vi "SVFA Zoom Coherent Output Power.vi"(0 "scaled signal X [EUx]":waveform(dbl)={"t0"=timestamp(0 s since 1904-01-01), "dt"=1e-05, "Y"=[]}, 1 "scaled signal Y [EUy]":waveform(dbl)={"t0"=timestamp(0 s since 1904-01-01), "dt"=1e-05, "Y"=[]}, 3 "zoom settings":T8={"frequency range"={"start frequency"=1000.0, "stop frequency"=2000.0}, "window"=1, "number of lines"=400, "% overlap"=0.0} {"% overlap" min=0.0 format="%.2f"; "number of lines" min=2; "window" items=["None ", "Hanning", "Hamming", "Blackman-Harris", "Exact Blackman", "Blackman", "Flat Top", "4 Term B-Harris ", "7 Term B-Harris", "Low Sidelobe"]; "frequency range"."stop frequency" min=0.0 format="%.2f"; "frequency range"."start frequency" min=0.0 format="%.2f"}, 4 "dB On (T)":bool=TRUE, 5 "error in (no error)":errorcluster, 7 "averaging parameters":T7={"averaging mode"=enum."No averaging", "weighting mode"=enum."Exponential", "number of averages"=10, "linear mode"=enum."One shot"} {"number of averages" min=1 step=1}, 9 "restart averaging (F)":bool) -> (10 "new spectrum available":bool, 11 "averaging done":bool, 12 "coherence":cluster{"f0":dbl, "df":dbl, "coherence":dbl[]} {"coherence" format="%.2p"; "df" format="%.2p"; "f0" format="%.2p"}, 13 "averages completed":dbl, 14 "coherent output power [dB EUy]":cluster{"f0":dbl, "df":dbl, "magnitude":dbl[]} {"magnitude" format="%.2p"; "df" format="%.2p"; "f0" format="%.2p"}, 15 "unit label":string, 18 "spectrum info":T1={"channel name"="", "description"="", "x-axis units"=1, "spectral info"={"spectrum type"=enum."Power [Magnitude^2]", "linear/dB"=enum."linear", "window"=0, "window size"=0, "FFT size"=0}, "engineering units"=0, "custom label"="", "dB reference [EU]"=0.0, "peak units"=enum."rms", "weighting filter"=0, "spectral density?"=FALSE, "unit label"="", "spectrum skewed?"=FALSE, "complimentary spectrum units"=enum."none"} {"x-axis units" items=["Time (s)"=0, "Frequency-CB (Hz)"=1, "Frequency-CPB (Hz)"=1248, "Frequency-Arbitrary (Hz)"=2357, "Quefrency (s)"=2, "Revolutions (rev)"=3, "Order"=4, "Speed (RPM)"=11, "Speed (rad/s)"=21, "Index"=65535]; "weighting filter" items=["Linear", "A-weighting", "B-weighting", "C-weighting", "ITU-R 468-4", "Dolby", "CCITT", "C-message", "Wb", "Wc", "Wd", "We", "Wf", "Wh", "Wj", "Wk", "Wm", "AES17 20 kHz lowpass", "AES17 40 kHz lowpass", "AES17 20 kHz highpass", "AES17 40 kHz highpass"]; "dB reference [EU]" format="%.2f"; "engineering units" items=["custom..."=0, "V"=1, "A"=21, "C"=30, "pC"=31, "s"=32, "-"=29, "Pa"=2, "N"=20, "g"=3, "m/s^2"=4, "m/s"=5, "m"=6, "mm/s"=12, "mm"=13, "micron/s"=14, "micron"=15, "in/s^2"=7, "in/s"=8, "in"=9, "mil/s"=10, "mil"=11, "rad/s^2"=16, "rad/s"=17, "rad"=18, "deg/s^2"=26, "deg/s"=27, "deg"=28, "RPM"=22, "cycle/s^2"=23, "Hz"=24, "cycle"=25, "strain"=19]; "spectral info"."window" items=["None "=0, "Hanning"=1, "Hamming"=2, "Blackman-Harris"=3, "Exact Blackman"=4, "Blackman"=5, "Flat Top"=6, "4 Term B-Harris "=7, "7 Term B-Harris"=8, "Low Sidelobe"=9, "Force - Exponential"=10, "Gaussian"=62]}, 19 "error out":errorcluster)   [LabVIEW 2017]
doc: "Computes the zoom coherent output power of <B>scaled signal X [EUx]</B>, <B>scaled signal Y [EUy]</B>, and <B>zoom settings</B>. Data accumulates each time the SVFA Zoom Coherent Output Power VI is called. However, it returns a new spectrum only when sufficient data accumulates. Indicators and subsequent processing should only be called when <B>new spectrum available</B> is TRUE.\n\nZoom coherent output power is typically an averaged measurement."
uses:
  <vilib>/addons/_NISVFA/_Shared subVIs/Controls/svc_Spectrum Info.ctl
  <vilib>/addons/_NISVFA/_Shared subVIs/Controls/svc_X-Axis Units.ctl
  <vilib>/addons/_NISVFA/_Shared subVIs/Controls/svc_Spectrum Type.ctl
  <vilib>/addons/_NISVFA/_Shared subVIs/Controls/svc_Engineering Units Text Ring.ctl
  <vilib>/addons/_NISVFA/_Shared subVIs/Controls/svc_Weighting Filter Text Ring.ctl
  <vilib>/addons/_NISVFA/_Shared subVIs/Controls/svc_Complimentary Spectrum Units.ctl
  <vilib>/addons/_NISVFA/_Shared subVIs/Common/svc_Get SV Channel Info.vi
  <vilib>/addons/_NISVFA/_Shared subVIs/Common/svc_Spectrum Units.vi
  <vilib>/addons/_NISVFA/_Shared subVIs/Common/svc_Get Weighting Enum and Labels.vi
  <vilib>/addons/_NISVFA/_Shared subVIs/Common/svc_Unit Label Lexical Class.vi
  <vilib>/addons/_NISVFA/_Shared subVIs/Common/svc_Engineering Units to Unit Label.vi
  <vilib>/addons/_NISVFA/_Shared subVIs/Common/svc_Format Value (DBL).vi
  <vilib>/addons/_NISVFA/_Shared subVIs/Common/svc_Channel Info to Spectrum Info.vi
  <vilib>/addons/_NISVFA/_Shared subVIs/Common/svc_Unit Label to Engineering Units.vi
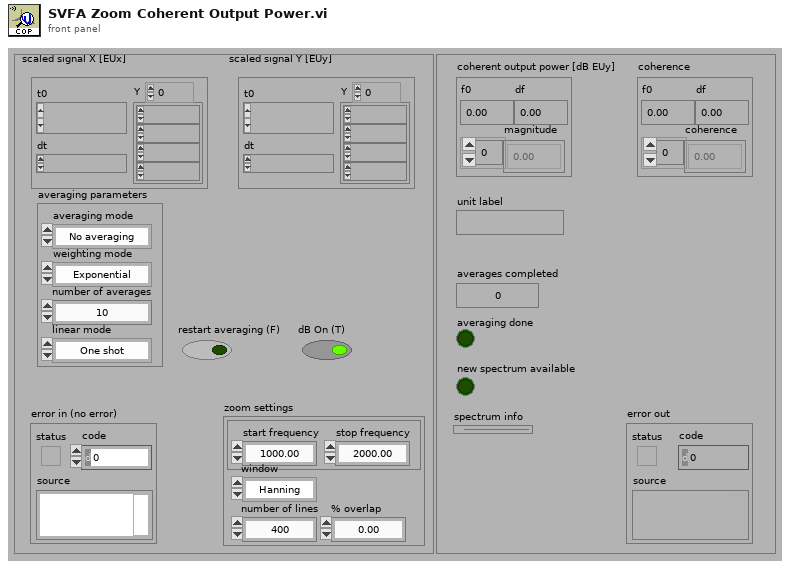
[diagram p1: front panel]
types:
  T1 = typedef "svc_Spectrum Info.ctl" = cluster{"channel name":string, "description":string, "x-axis units":T2, "spectral info":cluster{"spectrum type":T3, "linear/dB":enum16{"linear", "dB"}, "window":u16, "window size":i32, "FFT size":i32}, "engineering units":T4, "custom label":string, "dB reference [EU]":dbl, "peak units":enum16{"rms", "peak", "peak-peak"}, "weighting filter":T5, "spectral density?":bool, "unit label":string, "spectrum skewed?":bool, "complimentary spectrum units":T6}
  T2 = typedef "svc_X-Axis Units.ctl" = u16
  T3 = typedef "svc_Spectrum Type.ctl" = enum16{"FFT Spectrum [complex]", "Amplitude [Magnitude]", "Power [Magnitude^2]", "Cross Spectrum [complex]", "Frequency Response [Complex]"}
  T4 = typedef "svc_Engineering Units Text Ring.ctl" = u16
  T5 = typedef "svc_Weighting Filter Text Ring.ctl" = u16
  T6 = typedef "svc_Complimentary Spectrum Units.ctl" = enum16{"none", "radians", "degrees", "cycles", "imaginary"}
  T7 = cluster{"averaging mode":enum16{"No averaging", "Vector averaging", "RMS averaging", "Peak hold"}, "weighting mode":enum16{"Linear", "Exponential"}, "number of averages":u32, "linear mode":enum16{"One shot", "Auto restart"}}
  T8 = cluster{"frequency range":cluster{"start frequency":dbl, "stop frequency":dbl}, "window":u16, "number of lines":i32, "% overlap":dbl}
  T9 = enum16{"Restart processing", "Continue processing", "Skip processing"}
  T10 = enum16{"Cross spectrum", "Frequency response", "Coherent output power"}
  T11 = cluster{"zoom settings":cluster{"center frequency":dbl, "zoom":i32, "trim":dbl}, "FFT settings":cluster{"window":enum16{"None ", "Hanning", "Hamming", "Blackman-Harris", "Exact Blackman", "Blackman", "Flat Top", "4 Term B-Harris ", "7 Term B-Harris", "Low Sidelobe"}, "window size":i32, "FFT size":i32, "%overlap":dbl}}
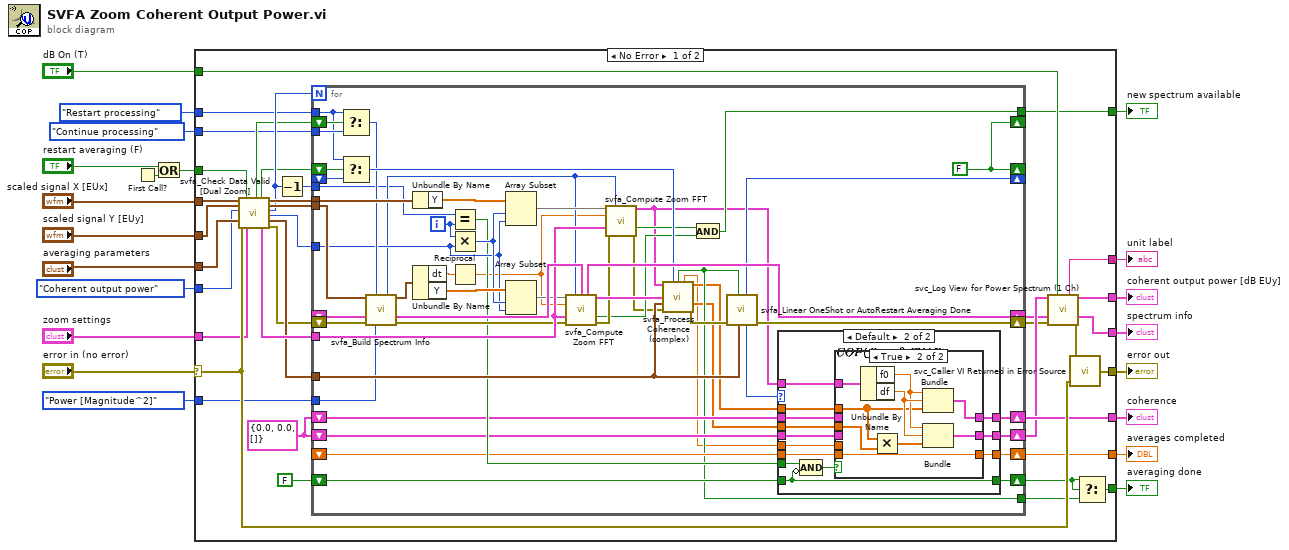
[diagram p0: block diagram]
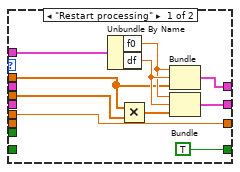
[diagram p2: hidden frame]
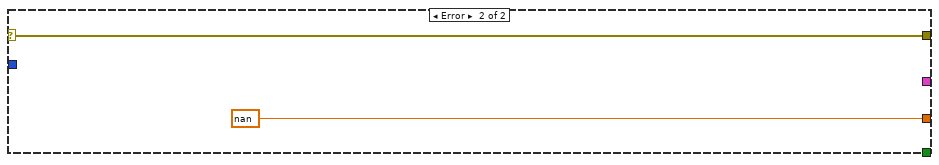
[diagram p4: hidden frame]
diagram:
  n1 = First Call?() -> (First Call?: T/F=w6:bool)
  n2 = Or(x="restart averaging (F)", y=w6) -> (x .or. y?=w5:bool)
  n3 = case shown="No Error" "error in (no error)" {
    selector: "error in (no error)" -> [w49 w148]
    tunnel: "averaging parameters" -> [w57 _]
    tunnel: "dB On (T)" -> [w56 _]
    tunnel: [w51 w148] -> w19
    tunnel: [w54 _] -> w18
    tunnel: "scaled signal X [EUx]" -> [w47 _]
    tunnel: "scaled signal Y [EUy]" -> [w58 _]
    tunnel: w5 -> [w48 _]
    tunnel: [w55 _] -> w13
    tunnel: [w23 nan ("averages completed")] -> w12
    tunnel: [w25 _] -> w11
    tunnel: "zoom settings" -> [w46 _]
    tunnel: [w41 _] -> w9
    tunnel: [w45 _] -> w8
    tunnel: [w52 _] -> w7
    tunnel: T10."Coherent output power" ("measurement") -> [w50 _]
    tunnel: T9."Restart processing" ("processing control") -> [w31 _]
    tunnel: T9."Continue processing" ("processing control") -> [w30 _]
    tunnel: svc_Spectrum_Type."Power [Magnitude^2]" ("spectrum type") -> [w28 _]
    frame No Error {
      w22 = cluster{"f0":dbl, "df":dbl, "Coherence":dbl[]} {"f0"=0.0, "df"=0.0, "Coherence"=[]}
      n4 = call <vilib>:"svfa_Check Data Valid [Dual Zoom].vi"("stimulus [X]"=w47, "response [Y]"=w58, "measurement"=w50, "averaging parameters"=w57, "error in (no error)"=w49, "restart averaging (F)"=w48, "zoom settings"=w46) -> ("reset processing"=w32:bool, "restart averaging"=w33:bool, "zoom FFT settings"=w44:T11, "dup stimulus [X]"=w38:waveform(dbl), "dup response [Y]"=w37:waveform(dbl), "iterations"=w35:i32, "maximum block size"=w29:i32, "dup averaging parameters"=w43:T7, "error out"=w36:errorcluster)  [unwired: 3 in, 1 out]
      n5 = Decrement(x=w35) -> (x-1=w34:i32)
      n6 = for {
        N: w35 -> [_]
        shift-left: _ -> [w102]
        shift-right: [w105] -> w40
        shift-left: w22 -> [w67]
        shift-right: [w69] -> w45
        tunnel: [w66] -> w24
        tunnel: [w79] -> w41
        tunnel: w43 -> [w111]
        shift-left: w22 -> [w68]
        shift-right: [w70] -> w42
        tunnel: w44 -> [w100]
        tunnel: w38 -> [w104]
        tunnel: w37 -> [w103]
        tunnel: w34 -> [w84]
        tunnel: w31 -> [w96]
        tunnel: w30 -> [w97]
        tunnel: w29 -> [w88]
        shift-right: [w110] -> w39
        shift-left: w36 -> [w101]
        shift-right: [w76] -> _
        shift-left: _ -> [w85]
        tunnel: w28 -> [w77]
        shift-right: [w74] -> w26
        shift-left: FALSE ("restart averaging") -> [w73]
        shift-right: [w72] -> w23
        shift-left: _ -> [w71]
        shift-right: [w59] -> _
        shift-left: w33 -> [w99]
        shift-right: [w59] -> _
        shift-left: w32 -> [w98]
        i -> [w83]
        w59 = FALSE ("restart averaging")
        n7 = Select(t=w96, s=w98, f=w97) -> (s? t:f=w92:T9)
        n8 = Select(t=w96, s=w99, f=w85) -> (s? t:f=w93:T9)
        n9 = call <vilib>:"svfa_Build Spectrum Info.vi"("scaled signal [EU]"=w103, "processing control"=w92, "spectrum info in"=w102, "error in (no error)"=w101, "spectrum type"=w77) -> ("dup processing control"=w86:T9, "dup scaled signal [EU]"=w108:waveform(dbl), "spectrum info out"=w107:T1, "error out"=w87:errorcluster)  [unwired: 7 in]
        n10 = Unbundle By Name ("Get Waveform Components")(w104) -> ("Y"=w95:dbl[])
        n11 = Unbundle By Name ("Get Waveform Components")(w108) -> ("dt"=w61:dbl, "Y"=w91:dbl[])
        n12 = Equal?(x=w84, y=w83) -> (x = y?=w75:bool)
        n13 = Multiply(x=w83, y=w88) -> (x*y=w89:i32)
        n14 = Reciprocal(x=w61) -> (1/x=w62:dbl)
        n15 = Array Subset(array=w95, index=w89, length=w88) -> (w94:dbl[])
        n16 = Array Subset(array=w91, index=w89, length=w88) -> (w90:dbl[])
        n17 = call <vilib>:"svfa_Compute Zoom FFT.vi"("x"=w90, "processing control"=w86, "spectrum info"=w107, "fs"=w62, "zoom FFT settings"=w100, "error in (no error)"=w87) -> ("spectrum info out"=w105:T1, "FFT spectrum"=w106:cluster{"f0":dbl, "df":dbl, "spectrum":cdb[]}, "spectrum ready"=w80:bool, "error out"=w82:errorcluster)  [unwired: 5 in, 1 out]
        n18 = call <vilib>:"svfa_Compute Zoom FFT.vi"("x"=w94, "processing control"=w86, "fs"=w62, "zoom FFT settings"=w100, "error in (no error)"=w82) -> ("FFT spectrum"=w65:cluster{"f0":dbl, "df":dbl, "spectrum":cdb[]}, "spectrum ready"=w81:bool, "error out"=w78:errorcluster)  [unwired: 6 in, 2 out]
        n19 = call <vilib>:"svfa_Process Coherence (complex).vi"("X FFT spectrum [Vrms]"=w65, "processing control"=w93, "Y FFT spectrum [Vrms]"=w106, "averaging parameters"=w111, "error in (no error)"=w78) -> ("averaging done"=w66:bool, "averages completed"=w60:dbl, "Coherence"=w64:dbl[], "<Gyy>"=w63:dbl[], "error out"=w109:errorcluster)  [unwired: 3 in, 3 out]
        n20 = And(x=w81, y=w80) -> (x .and. y?=w79:bool)
        n21 = call <vilib>:"svfa_Linear OneShot or AutoRestart Averaging Done.vi"("averaging parameters"=w111, "averaging done"=w66, "error in (no error)"=w109) -> ("error out"=w110:errorcluster, "processing control"=w76:T9)  [unwired: 7 in]
        n22 = case shown="Default" w76 {
          tunnel: w68 -> [_ w134]
          tunnel: [TRUE ("restart averaging") w129] -> w74
          tunnel: [w113 w133] -> w69
          tunnel: w73 -> [_ w129]
          tunnel: w75 -> [_ w132]
          tunnel: w67 -> [_ w131]
          tunnel: [w120 w128] -> w72
          tunnel: w71 -> [_ w127]
          tunnel: w60 -> [w120 w126]
          tunnel: [w112 w125] -> w70
          tunnel: w65 -> [w116 w124]
          tunnel: w64 -> [w115 w123]
          tunnel: w63 -> [w114 w122]
          frame "Restart processing" {
            n23 = Unbundle By Name(w116) -> ("f0"=w117:dbl, "df"=w118:dbl)
            n24 = Multiply(x=w115, y=w114) -> (x*y=w119:dbl[])
            n25 = Bundle("f0"=w117, "df"=w118, "Coherence"=w115) -> (w113:cluster{"f0":dbl, "df":dbl, "Coherence":dbl[]})  [unwired: 1 in]
            n26 = Bundle("f0"=w117, "df"=w118, w119) -> (w112:cluster{"f0":dbl, "df":dbl, dbl[]})  [unwired: 1 in]
          }
          frame Default {
            n27 = Compound Arithmetic op=AND(w132, invert w129) -> (w130:bool)
            n28 = case shown="True" w130 {
              tunnel: w134 -> [w135 _]
              tunnel: [w137 w139] -> w133
              tunnel: w131 -> [w137 _]
              tunnel: [w136 w146] -> w128
              tunnel: w127 -> [w136 _]
              tunnel: w126 -> [_ w146]
              tunnel: [w135 w138] -> w125
              tunnel: w124 -> [_ w142]
              tunnel: w123 -> [_ w141]
              tunnel: w122 -> [_ w140]
              frame False {
              }
              frame True {
                n29 = Unbundle By Name(w142) -> ("f0"=w143:dbl, "df"=w144:dbl)
                n30 = Multiply(x=w141, y=w140) -> (x*y=w145:dbl[])
                n31 = Bundle("f0"=w143, "df"=w144, "Coherence"=w141) -> (w139:cluster{"f0":dbl, "df":dbl, "Coherence":dbl[]})  [unwired: 1 in]
                n32 = Bundle("f0"=w143, "df"=w144, w145) -> (w138:cluster{"f0":dbl, "df":dbl, dbl[]})  [unwired: 1 in]
              }
            }
          }
        }
      }
      n33 = call <vilib>:"svc_Log View for Power Spectrum (1 Ch).vi"("power spectrum [dB EU]"=w42, "dB On (T)"=w56, "spectrum info"=w40, "error in (no error)"=w39) -> ("unit label"=w55:string, "power spectrum [dB EU]"=w54:cluster{"f0":dbl, "df":dbl, "magnitude":dbl[]}, "spectrum info out"=w52:T1, "error out"=w53:errorcluster)  [unwired: 8 in]
      n34 = call <vilib>:"svc_Caller VI Returned in Error Source.vi"("warning input to caller"=w49, "error in (no error)"=w53) -> ("error out"=w51:errorcluster)  [unwired: 3 in]
      n35 = Select(t=w26, s=w26, f=w24) -> (s? t:f=w25:bool)
    }
    frame Error {
    }
  }
  "error out" <- w19
  "coherent output power [dB EUy]" <- w18
  "unit label" <- w13
  "averages completed" <- w12
  "averaging done" <- w11
  "new spectrum available" <- w9
  "spectrum info" <- w7
  "coherence" <- w8
